vi "BotSpeak_Tiny.vi"(1 "URAPI":string) -> (2 "URAPI  2":string, 3 "SubsString":string, 4 "Tiny Lines":string[](array[string]))   [LabVIEW 2012]
panel:
  in  "Numeric":u8
  # "1st byte - length\n2nd byte - command\n3rd - nth byte values\n\nvalues are 2 bytes each\n\nNumber - is u16 ( hi byte first)\nOtherwise 8 bit source and 8 bit value\nIf MSB = 1, then it is an array\n\nsources:\n\n200 (C8) - TMR[#]\n201 (C9) - AI[#]\n202 (CA) - DIO[#]\n203 (CB) - PWM[#]\n204 (CC) - SERVO[#]\n\n220 (DC) - TMR[var]\n221 (DD) - AI[var]\n222 (DE) - DIO[var]\n223 (DF) - PWM[var]\n224 (E0) - SERVO[var]\n\n252 (FC) - \n253 (FD) - var[var]\n254 (FE) - \n255 (FF) - var#"
  # "a.. abort\nd.. dump\n+ (x2B).. add\n-*/\n\ng (x67)..get\nG (x47)..goto\nI.. (x49) if\n   < x3C\ni.. not if\nP..ping\nr (x72)..run\nd..debug\nR..run and wait\ns (x73)..script\nE (x45).. end script\ne ... go to ScriptSize\n= (x3D)..set\nW (x57)..wait (ms)\nw (x77)..wait (µs)"
  # "DIO 1,1 - raises port 1 high\nDIO 1 - retrieves the status of DIO 1\nSERVO 1,1.5 - sets servo 1 to 1.5 msec (-1 turns off)\nABORT - stops\nDUMP - gives state of all DIO lines in 2 numbers\nAI 0 - replies with value of channel 0\nAO 0,2.5 - sets PWM out to 50%\nSET test,1.2 - sets variable test to 1.2\nGET test - gets value of variable test\nPING - returns version number\nTIMER 1,"
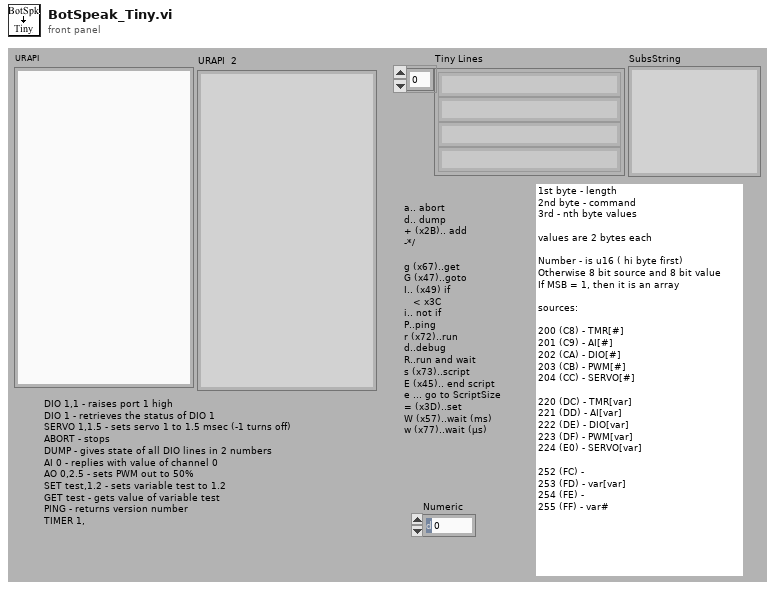
[diagram p1: front panel]
types:
  T1 = cluster{"upper limit":dbl, "lower limit":dbl, "scale":dbl}[]
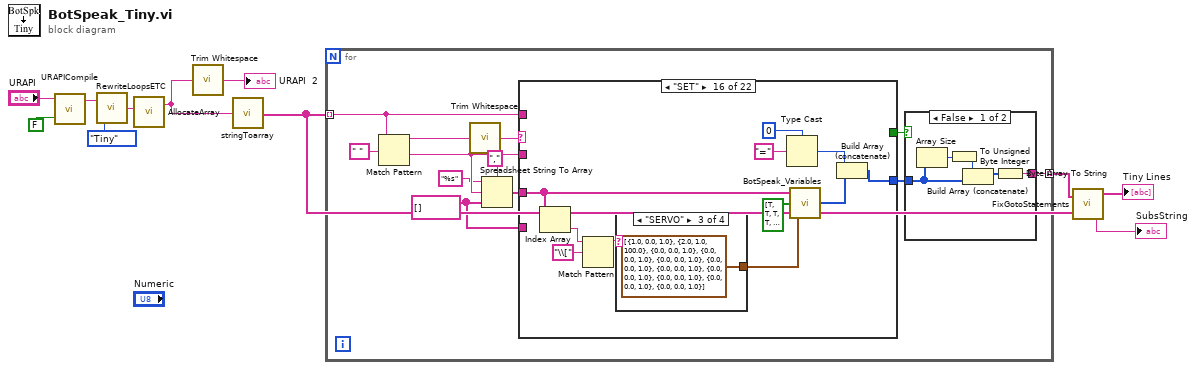
[diagram p0: block diagram]
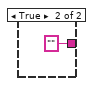
[diagram p2: hidden frame]
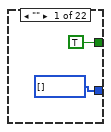
[diagram p3: hidden frame]
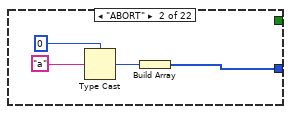
[diagram p4: hidden frame]
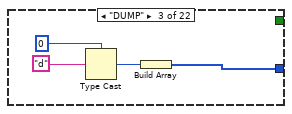
[diagram p5: hidden frame]
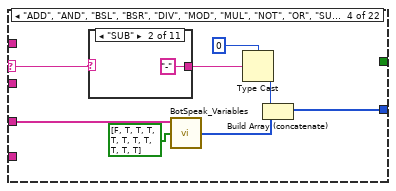
[diagram p6: hidden frame]
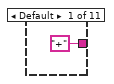
[diagram p7: hidden frame]
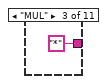
[diagram p8: hidden frame]
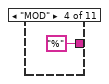
[diagram p9: hidden frame]
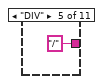
[diagram p10: hidden frame]
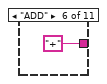
[diagram p11: hidden frame]
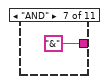
[diagram p12: hidden frame]
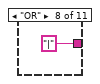
[diagram p13: hidden frame]
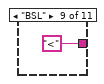
[diagram p14: hidden frame]
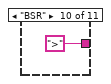
[diagram p15: hidden frame]
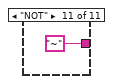
[diagram p16: hidden frame]
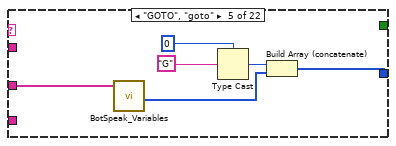
[diagram p17: hidden frame]
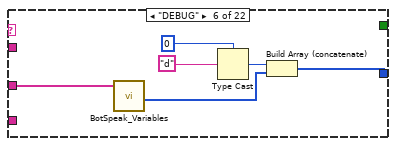
[diagram p18: hidden frame]
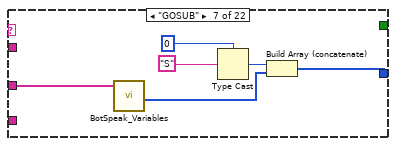
[diagram p19: hidden frame]
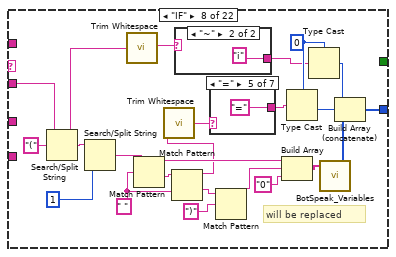
[diagram p20: hidden frame]
diagram:
  n1 = call <userlib>:"URAPICompile.vi"("Comments?"=FALSE, "Script"="URAPI") -> ("trimmed script"=w10:string)
  n2 = call <userlib>:"RewriteLoopsETC.vi"("Type"=enum16{"Tiny", "BotSpeak"}."Tiny", "URAPI in"=w10) -> ("URAPI out"=w6:string)
  n3 = call <userlib>:"AllocateArray.vi"("URAPI in"=w6) -> ("URAPI out"=w5:string)  [unwired: 2 in]
  n4 = call <vilib>:"Trim Whitespace.vi"("string"=w5) -> ("trimmed string"=→"URAPI  2":string)  [unwired: 1 in]
  n5 = call <userlib>:"stringToarray.vi"("String"=w5) -> ("Array"=w4:string[])
  n6 = for {
    tunnel: [w16] -> w8 mode=indexing
    tunnel: w4 -> [w12] mode=indexing
    w14 = string[] []
    n7 = Match Pattern(string=w12, regular expression=" ") -> (before substring=w22:string, after substring=w20:string)  [unwired: 1 in, 2 out]
    n8 = call <vilib>:"Trim Whitespace.vi"("string"=w22) -> ("trimmed string"=w21:string)  [unwired: 1 in]
    n9 = Spreadsheet String To Array(delimiter (Tab)=",", format string="%s", spreadsheet string=w20, array type (2D Dbl)=w14) -> (array=w18:string[])
    n10 = case shown="\"SET\"" w21 {
      selector: w21 -> [_ _ _ w41 _ _ _ _ _ _ _ _ _ _ _ _ _ _ _ _ _ _]
      tunnel: w12 -> [_ _ _ _ _ _ _ _ _ _ _ _ _ _ _ _ _ _ _ _ _ w217]
      tunnel: w20 -> [_ _ _ _ _ _ _ w98 _ _ _ w135 _ _ _ _ _ _ _ _ _ _]
      tunnel: w18 -> [_ _ _ w43 w60 w66 w72 _ _ w114 w120 w129 _ _ w150 w159 w175 w181 w188 w210 w216 _]
      tunnel: [u8[] [] ("unsigned byte array") w32 w36 w45 w61 w67 w73 w99 w110 w115 w121 w136 w140 w144 w151 w163 w176 w183 w193 w212 w215 w218] -> w17
      tunnel: [TRUE _ _ _ _ _ _ _ _ _ _ _ _ _ _ _ _ _ _ _ _ _] -> w15
      tunnel: w14 -> [_ _ _ _ _ _ _ _ _ _ _ _ _ _ _ _ _ _ _ _ _ _]
      frame "" {
      }
      frame "ABORT" {
        n11 = Type Cast(type=u8 0, x="a" ("delimiter (Tab)")) -> (*(type *) &x=w33:u8)
        n12 = Build Array(w33) -> (w32:u8[])
      }
      frame "DUMP" {
        n13 = Type Cast(type=u8 0, x="d" ("delimiter (Tab)")) -> (*(type *) &x=w37:u8)
        n14 = Build Array(w37) -> (w36:u8[])
      }
      frame "ADD", "AND", "BSL", "BSR", "DIV", "MOD", "MUL", "NOT", "OR", "SUB" {
        n15 = case shown="\"SUB\"" w41 {
          tunnel: ["+" ("delimiter (Tab)") "-" ("delimiter (Tab)") "*" ("delimiter (Tab)") "%" ("delimiter (Tab)") "/" ("delimiter (Tab)") "+" ("delimiter (Tab)") "&" ("delimiter (Tab)") "|" ("delimiter (Tab)") "<" ("delimiter (Tab)") ">" ("delimiter (Tab)") "~" ("delimiter (Tab)")] -> w40
          frame Default {
          }
          frame "SUB" {
          }
          frame "MUL" {
          }
          frame "MOD" {
          }
          frame "DIV" {
          }
          frame "ADD" {
          }
          frame "AND" {
          }
          frame "OR" {
          }
          frame "BSL" {
          }
          frame "BSR" {
          }
          frame "NOT" {
          }
        }
        n16 = call <userlib>:"BotSpeak_Variables.vi"("Var #?"=bool[] [FALSE, TRUE, TRUE, TRUE, TRUE, TRUE, TRUE, TRUE, TRUE, TRUE, TRUE] ("Value of?"), "Variables"=w43) -> ("Binary out"=w46:u8[])  [unwired: 1 in]
        n17 = Type Cast(type=u8 0, x=w40) -> (*(type *) &x=w44:u8)
        n18 = Build Array (concatenate)(w44, w46) -> (w45:u8[])
      }
      frame "GOTO", "goto" {
        n19 = call <userlib>:"BotSpeak_Variables.vi"("Variables"=w60) -> ("Binary out"=w59:u8[])  [unwired: 2 in]
        n20 = Type Cast(type=u8 0, x="G" ("delimiter (Tab)")) -> (*(type *) &x=w62:u8)
        n21 = Build Array (concatenate)(w62, w59) -> (w61:u8[])
      }
      frame "DEBUG" {
        n22 = call <userlib>:"BotSpeak_Variables.vi"("Variables"=w66) -> ("Binary out"=w65:u8[])  [unwired: 2 in]
        n23 = Type Cast(type=u8 0, x="d" ("delimiter (Tab)")) -> (*(type *) &x=w68:u8)
        n24 = Build Array (concatenate)(w68, w65) -> (w67:u8[])
      }
      frame "GOSUB" {
        n25 = call <userlib>:"BotSpeak_Variables.vi"("Variables"=w72) -> ("Binary out"=w71:u8[])  [unwired: 2 in]
        n26 = Type Cast(type=u8 0, x="S" ("delimiter (Tab)")) -> (*(type *) &x=w74:u8)
        n27 = Build Array (concatenate)(w74, w71) -> (w73:u8[])
      }
      frame "IF" {
        w95 = " " ("regular expression")
        w90 = u8 0
        # "will be replaced"
        n28 = Search/Split String(string=w98, search string/char (-)="(" ("regular expression")) -> (substring before match=w85:string, match + rest of string=w80:string)  [unwired: 1 in, 1 out]
        n29 = Search/Split String(string=w80, offset (0)=1) -> (match + rest of string=w78:string)  [unwired: 1 in, 2 out]
        n30 = call <vilib>:"Trim Whitespace.vi"("string"=w85) -> ("trimmed string"=w84:string)  [unwired: 1 in]
        n31 = Match Pattern(string=w78, regular expression=w95) -> (before substring=w91:string, after substring=w96:string)  [unwired: 1 in, 2 out]
        n32 = Match Pattern(string=w96, regular expression=w95) -> (before substring=w89:string, after substring=w94:string)  [unwired: 1 in, 2 out]
        n33 = call <vilib>:"Trim Whitespace.vi"("string"=w89) -> ("trimmed string"=w88:string)  [unwired: 1 in]
        n34 = case shown="\"~\"" w84 {
          tunnel: ["I" ("delimiter (Tab)") "i" ("delimiter (Tab)")] -> w83
          frame Default {
          }
          frame "~" {
          }
        }
        n35 = case shown="\"=\"" w88 {
          tunnel: ["<" ("delimiter (Tab)") "<" ("delimiter (Tab)") ">" ("delimiter (Tab)") "!" ("delimiter (Tab)") "=" ("delimiter (Tab)") "G" ("delimiter (Tab)") "L" ("delimiter (Tab)")] -> w87
          frame Default {
          }
          frame "<" {
          }
          frame ">" {
          }
          frame "!=", "<>" {
          }
          frame "=" {
          }
          frame ">=" {
          }
          frame "<=" {
          }
        }
        n36 = Match Pattern(string=w94, regular expression=")") -> (before substring=w92:string)  [unwired: 1 in, 3 out]
        n37 = Build Array(w91, w92, "0" ("regular expression")) -> (w82:string[])
        n38 = Type Cast(type=w90, x=w87) -> (*(type *) &x=w86:u8)
        n39 = Type Cast(type=w90, x=w83) -> (*(type *) &x=w100:u8)
        n40 = call <userlib>:"BotSpeak_Variables.vi"("Variables"=w82) -> ("Binary out"=w81:u8[])  [unwired: 2 in]
        n41 = Build Array (concatenate)(w100, w86, w81) -> (w99:u8[])
      }
      frame "PING" {
        n42 = Type Cast(type=u8 0, x="P" ("delimiter (Tab)")) -> (*(type *) &x=w111:u8)
        n43 = Build Array(w111) -> (w110:u8[])
      }
      frame "RUN" {
        n44 = call <userlib>:"BotSpeak_Variables.vi"("Variables"=w114) -> ("Binary out"=w116:u8[])  [unwired: 2 in]
        n45 = Type Cast(type=u8 0, x="r" ("delimiter (Tab)")) -> (*(type *) &x=w117:u8)
        n46 = Build Array (concatenate)(w117, w116) -> (w115:u8[])
      }
      frame "RUN&WAIT" {
        n47 = call <userlib>:"BotSpeak_Variables.vi"("Variables"=w120) -> ("Binary out"=w122:u8[])  [unwired: 2 in]
        n48 = Type Cast(type=u8 0, x="R" ("delimiter (Tab)")) -> (*(type *) &x=w123:u8)
        n49 = Build Array (concatenate)(w123, w122) -> (w121:u8[])
      }
      frame "SCRIPT" {
        n50 = Match Pattern(string=w135, regular expression="," ("delimiter (Tab)")) -> (after substring=w131:string)  [unwired: 1 in, 3 out]
        n51 = Match Pattern(string=w131, regular expression="," ("delimiter (Tab)")) -> (after substring=w130:string)  [unwired: 1 in, 3 out]
        n52 = Array Subset(array=w129, length=2) -> (w127:string[])  [unwired: 1 in]
        n53 = call <userlib>:"BotSpeak_Variables.vi"("Variables"=w127) -> ("Binary out"=w126:u8[])  [unwired: 2 in]
        n54 = String To Byte Array(string=w130) -> (unsigned byte array=w133:u8[])
        n55 = Type Cast(type=u8 0, x="s" ("delimiter (Tab)")) -> (*(type *) &x=w137:u8)
        n56 = Build Array (concatenate)(w137, w126, w133) -> (w136:u8[])
      }
      frame "ENDSCRIPT" {
        n57 = Type Cast(type=u8 0, x="E" ("delimiter (Tab)")) -> (*(type *) &x=w141:u8)
        n58 = Build Array(w141) -> (w140:u8[])
      }
      frame "END", "end" {
        n59 = Type Cast(type=u8 0, x="e" ("delimiter (Tab)")) -> (*(type *) &x=w145:u8)
        n60 = Build Array(w145) -> (w144:u8[])
      }
      frame "SERVO" {
        n61 = Type Cast(type=u8 0, x="S" ("delimiter (Tab)")) -> (*(type *) &x=w152:u8)
        n62 = call <userlib>:"BotSpeak_Variables.vi"("Scaling"=T1 [{"upper limit"=0.0, "lower limit"=0.0, "scale"=0.0}, {"upper limit"=3.0, "lower limit"=0.0, "scale"=180.0}], "Variables"=w150) -> ("Binary out"=w148:u8[])  [unwired: 1 in]
        n63 = Build Array (concatenate)(w152, w148) -> (w151:u8[])
      }
      frame "SET" {
        n64 = Index Array(array=w159) -> (element=w158:string)  [unwired: 1 in]
        n65 = Match Pattern(string=w158, regular expression="\\[") -> (before substring=w156:string)  [unwired: 1 in, 3 out]
        n66 = case shown="\"SERVO\"" w156 {
          tunnel: [T1 [{"upper limit"=0.0, "lower limit"=0.0, "scale"=1.0}, {"upper limit"=2.0, "lower limit"=1.0, "scale"=100.0}, {"upper limit"=0.0, "lower limit"=0.0, "scale"=1.0}, {"upper limit"=0.0, "lower limit"=0.0, "scale"=1.0}, {"upper limit"=0.0, "lower limit"=0.0, "scale"=1.0}, {"upper limit"=0.0, "lower limit"=0.0, "scale"=1.0}, {"upper limit"=0.0, "lower limit"=0.0, "scale"=1.0}, {"upper limit"=0.0, "lower limit"=0.0, "scale"=1.0}, {"upper limit"=0.0, "lower limit"=0.0, "scale"=1.0}, {"upper limit"=0.0, "lower limit"=0.0, "scale"=1.0}, {"upper limit"=0.0, "lower limit"=0.0, "scale"=1.0}] ("Scaling") T1 [{"upper limit"=1.0, "lower limit"=0.0, "scale"=1.0}, {"upper limit"=100.0, "lower limit"=0.0, "scale"=100.0}, {"upper limit"=1.0, "lower limit"=0.0, "scale"=1.0}, {"upper limit"=0.0, "lower limit"=0.0, "scale"=1.0}, {"upper limit"=0.0, "lower limit"=0.0, "scale"=1.0}, {"upper limit"=0.0, "lower limit"=0.0, "scale"=1.0}, {"upper limit"=0.0, "lower limit"=0.0, "scale"=1.0}, {"upper limit"=0.0, "lower limit"=0.0, "scale"=1.0}, {"upper limit"=0.0, "lower limit"=0.0, "scale"=1.0}, {"upper limit"=0.0, "lower limit"=0.0, "scale"=1.0}, {"upper limit"=0.0, "lower limit"=0.0, "scale"=1.0}] ("Scaling") T1 [{"upper limit"=1.0, "lower limit"=0.0, "scale"=1.0}, {"upper limit"=2.0, "lower limit"=1.0, "scale"=100.0}, {"upper limit"=0.0, "lower limit"=0.0, "scale"=1.0}, {"upper limit"=0.0, "lower limit"=0.0, "scale"=1.0}, {"upper limit"=0.0, "lower limit"=0.0, "scale"=1.0}, {"upper limit"=0.0, "lower limit"=0.0, "scale"=1.0}, {"upper limit"=0.0, "lower limit"=0.0, "scale"=1.0}, {"upper limit"=0.0, "lower limit"=0.0, "scale"=1.0}, {"upper limit"=0.0, "lower limit"=0.0, "scale"=1.0}, {"upper limit"=0.0, "lower limit"=0.0, "scale"=1.0}, {"upper limit"=0.0, "lower limit"=0.0, "scale"=1.0}] ("Scaling") T1 [{"upper limit"=0.0, "lower limit"=0.0, "scale"=1.0}, {"upper limit"=1.0, "lower limit"=0.0, "scale"=1.0}, {"upper limit"=0.0, "lower limit"=0.0, "scale"=1.0}, {"upper limit"=0.0, "lower limit"=0.0, "scale"=1.0}, {"upper limit"=0.0, "lower limit"=0.0, "scale"=1.0}, {"upper limit"=0.0, "lower limit"=0.0, "scale"=1.0}, {"upper limit"=0.0, "lower limit"=0.0, "scale"=1.0}, {"upper limit"=0.0, "lower limit"=0.0, "scale"=1.0}, {"upper limit"=0.0, "lower limit"=0.0, "scale"=1.0}, {"upper limit"=0.0, "lower limit"=0.0, "scale"=1.0}, {"upper limit"=0.0, "lower limit"=0.0, "scale"=1.0}] ("Scaling")] -> w155
          frame Default {
          }
          frame "PWM" {
          }
          frame "SERVO" {
          }
          frame "DIO" {
          }
        }
        n67 = Type Cast(type=u8 0, x="=" ("delimiter (Tab)")) -> (*(type *) &x=w162:u8)
        n68 = call <userlib>:"BotSpeak_Variables.vi"("Scaling"=w155, "Var #?"=bool[] [TRUE, TRUE, TRUE, TRUE, TRUE, TRUE, TRUE, TRUE, TRUE, TRUE, TRUE] ("Value of?"), "Variables"=w159) -> ("Binary out"=w160:u8[])
        n69 = Build Array (concatenate)(w162, w160) -> (w163:u8[])
      }
      frame "SYSTEM" {
        n70 = call <userlib>:"BotSpeak_Variables.vi"("Var #?"=bool[] [TRUE, TRUE, TRUE, TRUE, TRUE, TRUE, TRUE, TRUE, TRUE, TRUE, TRUE] ("Value of?"), "Variables"=w175) -> ("Binary out"=w172:u8[])  [unwired: 1 in]
        n71 = Array Size(array=w172) -> (size(s)=w171:i32)
        n72 = Type Cast(type=u8 0, x="!" ("delimiter (Tab)")) -> (*(type *) &x=w173:u8)
        n73 = To Unsigned Byte Integer(number=w171) -> (unsigned 8bit integer=w170:u8)
        n74 = Build Array (concatenate)(w173, w170, w172) -> (w176:u8[])
      }
      frame "GET" {
        n75 = Type Cast(type=u8 0, x="g" ("delimiter (Tab)")) -> (*(type *) &x=w182:u8)
        n76 = call <userlib>:"BotSpeak_Variables.vi"("Var #?"=bool[] [TRUE, TRUE, TRUE, TRUE, TRUE, TRUE, TRUE, TRUE, TRUE, TRUE, TRUE] ("Value of?"), "Variables"=w181) -> ("Binary out"=w179:u8[])  [unwired: 1 in]
        n77 = Build Array (concatenate)(w182, w179) -> (w183:u8[])
      }
      frame "WAIT" {
        n78 = Index Array(array=w188) -> (element=w191:string)  [unwired: 1 in]
        n79 = Scan From String(input string=w191) -> (error out=w190:errorcluster, output 1=w189:dbl)  [unwired: 4 in, 2 out]
        n80 = case shown="No Error" w190 {
          tunnel: [w197 "W" ("delimiter (Tab)")] -> w192
          tunnel: w189 -> [w201 _]
          tunnel: w188 -> [_ _]
          tunnel: [w196 T1 [{"upper limit"=0.0, "lower limit"=0.0, "scale"=1.0}] ("Scaling")] -> w186
          frame No Error {
            n81 = Absolute Value(x=w201) -> (abs(x)=w200:dbl)
            n82 = Less?(x=w200, y=0.01) -> (x < y?=w198:bool)
            n83 = case shown="True" w198 {
              tunnel: ["w" ("delimiter (Tab)") "W" ("delimiter (Tab)")] -> w197
              tunnel: [T1 [{"upper limit"=0.0, "lower limit"=0.0, "scale"=1000000.0}] ("Scaling") T1 [{"upper limit"=0.0, "lower limit"=0.0, "scale"=1000.0}] ("Scaling")] -> w196
              frame True {
              }
              frame False {
              }
            }
          }
          frame Error {
            # "variable for wait time\n(in msec)"
          }
        }
        n84 = Type Cast(type=u8 0, x=w192) -> (*(type *) &x=w194:u8)
        n85 = call <userlib>:"BotSpeak_Variables.vi"("Scaling"=w186, "Variables"=w188) -> ("Binary out"=w187:u8[])  [unwired: 1 in]
        n86 = Build Array (concatenate)(w194, w187) -> (w193:u8[])
      }
      frame "WAITµs" {
        n87 = call <userlib>:"BotSpeak_Variables.vi"("Scaling"=T1 [{"upper limit"=0.0, "lower limit"=0.0, "scale"=1.0}], "Variables"=w210) -> ("Binary out"=w208:u8[])  [unwired: 1 in]
        n88 = Type Cast(type=u8 0, x="w" ("delimiter (Tab)")) -> (*(type *) &x=w213:u8)
        n89 = Build Array (concatenate)(w213, w208) -> (w212:u8[])
      }
      frame "convert" {
        n90 = call <userlib>:"BotSpeak_Variables.vi"("Variables"=w216) -> ("Binary out"=w215:u8[])  [unwired: 2 in]
      }
      frame Default {
        n91 = String To Byte Array(string=w217) -> (unsigned byte array=w218:u8[])
      }
    }
    n92 = case shown="False" w15 {
      tunnel: w17 -> [w26 _]
      tunnel: [w28 "" ("string")] -> w16
      frame False {
        n93 = Array Size(array=w26) -> (size(s)=w27:i32)
        n94 = To Unsigned Byte Integer(number=w27) -> (unsigned 8bit integer=w24:u8)
        n95 = Build Array (concatenate)(w24, w26) -> (w25:u8[])
        n96 = Byte Array To String(unsigned byte array=w25) -> (string=w28:string)
      }
      frame True {
      }
    }
  }
  n97 = call <userlib>:"FixGotoStatements.vi"("URAPI LInes"=w4, "Tiny Lines"=w8) -> ("SubsString"=→"SubsString":string, "Tiny Fixed"=→"Tiny Lines":string[])  [unwired: 1 out]
